vi "Initialize Joystick.vi"(8 "error in (no error)":errorcluster) -> (0 "error out":errorcluster, 1 "input devices count":i32, 2 "device name":string, 3 "joystick info":T1(array[cluster]), 5 "Can't find device":bool)   [LabVIEW 2014, in "Joystick Fight Simulator.lvlib"]
doc: "Initialize joystick, list devices and looking for one with string \"2-axis\" in device name. That in my case when using LogiLing converter from gameport to usb."
uses:
  Joystick Fight Simulator.lvlib
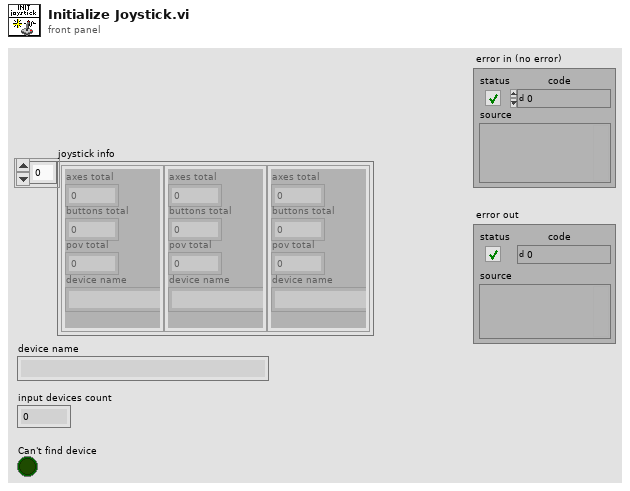
[diagram p1: front panel]
types:
  T1 = cluster{"axes total":u32, "buttons total":u32, "pov total":u32, "device name":string}[]
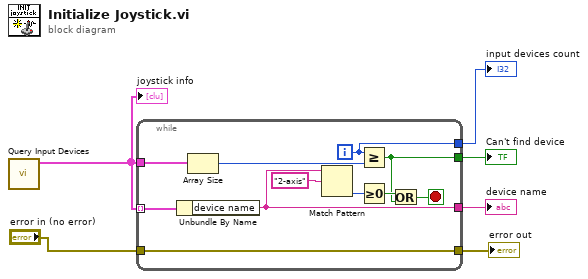
[diagram p0: block diagram]
diagram:
  n1 = call <vilib>:"Query Input Devices.vi"() -> ("joystick info"=w6:T1)  [unwired: 8 in, 3 out]
  "joystick info" <- w6
  n2 = while {
    tunnel: w6 -> [w17] mode=indexing
    tunnel: w6 -> [w14]
    tunnel: [w10] -> w5
    tunnel: [w9] -> w3
    tunnel: [w8] -> w4
    tunnel: "error in (no error)" -> [w7]
    tunnel: [w7] -> w1
    i -> [w8]
    stop <- w11 stop-if-true
    n3 = Unbundle By Name(w17) -> ("device name"=w9:string)
    n4 = Array Size(array=w14) -> (size(s)=w13:i32)
    n5 = Match Pattern(string=w9, regular expression="2-axis") -> (offset past match=w15:i32)  [unwired: 1 in, 3 out]
    n6 = Greater Or Equal?(x=w8, y=w13) -> (x >= y?=w10:bool)
    n7 = Greater Or Equal To 0?(x=w15) -> (x >= 0?=w12:bool)
    n8 = Or(x=w12, y=w10) -> (x .or. y?=w11:bool)
  }
  "Can't find device" <- w5
  "device name" <- w3
  "input devices count" <- w4
  "error out" <- w1
